vi "Check Version for Match.vi"(10 "Version to Match":string, 11 "PPL Path":path) -> (1 "Matches Version":bool, 2 "Version String":string)   [LabVIEW 2019]
uses:
  <vilib>/regexp/Match Regular Expression.xnode
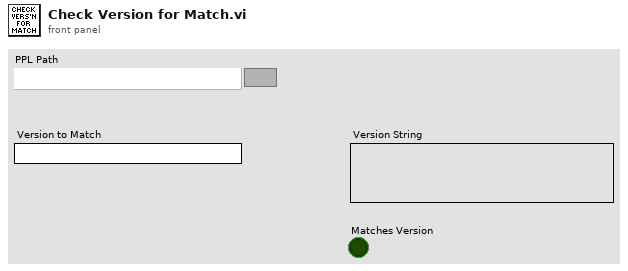
[diagram p1: front panel]
types:
  T1 = cluster{"Version":string, "Commit Reference":string}
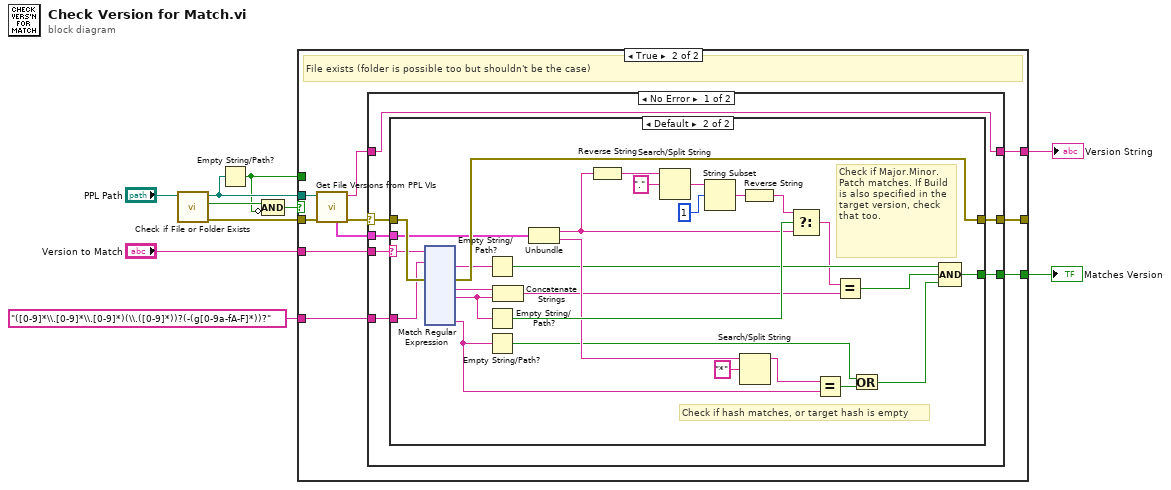
[diagram p0: block diagram]
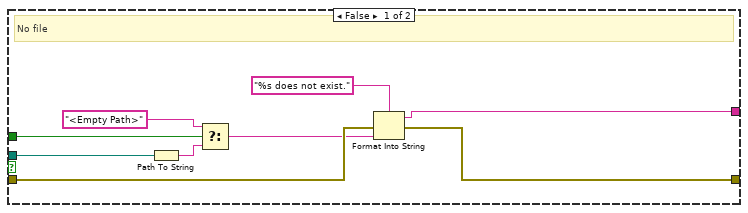
[diagram p2: hidden frame]
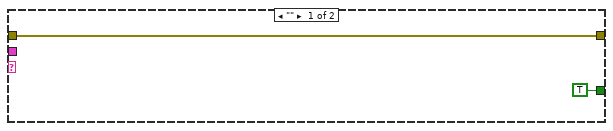
[diagram p3: hidden frame]
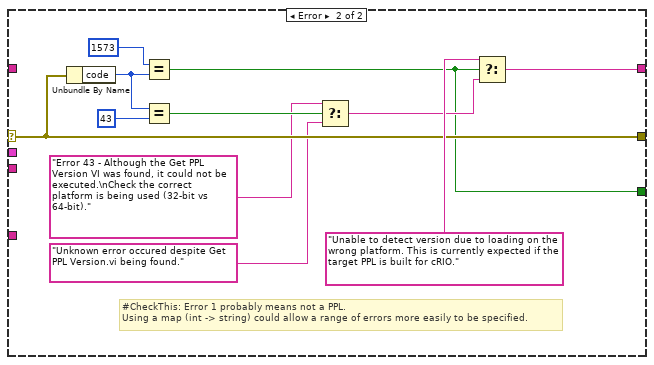
[diagram p4: hidden frame]
diagram:
  n1 = call <vilib>:"Check if File or Folder Exists.vi"("path"="PPL Path") -> ("error out"=w9:errorcluster, "file or folder exists?"=w5:bool, "dup path"=w6:path)  [unwired: 8 in]
  n2 = Empty String/Path?(string/path=w6) -> (empty?=w3:bool)
  n3 = Compound Arithmetic op=AND(w5, invert w3) -> (w4:bool)
  n4 = case shown="True" w4 {
    tunnel: "([0-9]*\\.[0-9]*\\.[0-9]*)(\\.([0-9]*))?(-(g[0-9a-fA-F]*))?" ("regular expression") -> [_ w29]
    tunnel: "Version to Match" -> [_ w28]
    tunnel: w9 -> [w19 w26]
    tunnel: w6 -> [w15 w25]
    tunnel: [_ w24] -> w8
    tunnel: [w11 w23] -> _
    tunnel: [w17 w22] -> w7
    tunnel: w3 -> [w16 _]
    frame False {
      # "No file"
      n5 = Path To String(path=w15) -> (string=w13:string)
      n6 = Select(t="<Empty Path>", s=w16, f=w13) -> (s? t:f=w12:string)
      n7 = Format Into String(format string="%s does not exist." ("Text to Write"), error in=w19, w12) -> (resulting string=w17:string, error out=w11:errorcluster)  [unwired: 1 in]
    }
    frame True {
      # "File exists (folder is possible too but shouldn't be the case)"
      n8 = call "Get File Versions from PPL VIs.vi"("error in (no error)"=w26, "Path"=w25) -> ("error IO"=w20:errorcluster, "Version with Hash"=w21:string, "Version Cluster"=w27:T1)  [unwired: 5 in, 2 out]
      n9 = case shown="No Error" w20 {
        selector: w20 -> [w31 w196]
        tunnel: w29 -> [w36 _]
        tunnel: w28 -> [w35 _]
        tunnel: w27 -> [w34 _]
        tunnel: [w33 w187] -> w24
        tunnel: [w32 w196] -> w23
        tunnel: [w30 w188] -> w22
        tunnel: w21 -> [w30 _]
        frame No Error {
          n10 = case shown="Default" w35 {
            selector: w35 -> [_ w40]
            tunnel: w31 -> [w37 w64]
            tunnel: w36 -> [_ w63]
            tunnel: [TRUE w41] -> w33
            tunnel: w34 -> [_ w39]
            tunnel: [w37 w66] -> w32
            frame "" {
            }
            frame Default {
              # "Check if Major.Minor.Patch matches. If Build is also specified in the target version, check that too."
              # "Check if hash matches, or target hash is empty"
              n11 = xnode "Match Regular Expression"("input string"=w40, "regular expression"=w63, "error in"=w64) -> ("after match"=w62:string, "error out"=w66:errorcluster, "submatch 1"=w60:string, "submatch 2"=w61:string, "submatch 5"=w54:string)  [unwired: 3 in, 5 out]
              n12 = Empty String/Path?(string/path=w62) -> (empty?=w50:bool)
              n13 = Empty String/Path?(string/path=w61) -> (empty?=w65:bool)
              n14 = Empty String/Path?(string/path=w54) -> (empty?=w43:bool)
              n15 = Concatenate Strings(w60, w61) -> (w46:string)
              n16 = Unbundle(w39) -> ("Version"=w48:string, "Commit Reference"=w53:string)
              n17 = Reverse String(1:w48) -> (0:w59:string)
              n18 = Search/Split String(string=w59, search string/char (-)=".") -> (match + rest of string=w57:string)  [unwired: 1 in, 2 out]
              n19 = String Subset(string=w57, offset (0)=1) -> (substring=w55:string)  [unwired: 1 in]
              n20 = Search/Split String(string=w53, search string/char (-)="*") -> (substring before match=w51:string)  [unwired: 1 in, 2 out]
              n21 = Reverse String(1:w55) -> (0:w49:string)
              n22 = Select(t=w49, s=w65, f=w48) -> (s? t:f=w47:string)
              n23 = Equal?(x=w51, y=w54) -> (x = y?=w44:bool)
              n24 = Equal?(x=w47, y=w46) -> (x = y?=w45:bool)
              n25 = Or(x=w43, y=w44) -> (x .or. y?=w42:bool)
              n26 = Compound Arithmetic op=AND(w50, w45, w42) -> (w41:bool)
            }
          }
        }
        frame Error {
          # "#CheckThis: Error 1 probably means not a PPL.\nUsing a map (int -> string) could allow a range of errors more easily to be specified."
          n27 = Unbundle By Name(w196) -> ("code"=w191:i32)
          n28 = Equal?(x=1573, y=w191) -> (x = y?=w187:bool)
          n29 = Equal?(x=w191, y=43 ("x")) -> (x = y?=w194:bool)
          n30 = Select(t="Error 43 - Although the Get PPL Version VI was found, it could not be executed.\nCheck the correct platform is being used (32-bit vs 64-bit).", s=w194, f="Unknown error occured despite Get PPL Version.vi being found.") -> (s? t:f=w189:string)
          n31 = Select(t="Unable to detect version due to loading on the wrong platform. This is currently expected if the target PPL is built for cRIO.", s=w187, f=w189) -> (s? t:f=w188:string)
        }
      }
    }
  }
  "Matches Version" <- w8
  "Version String" <- w7
